vi "is absolute path.vi"(11 "path":string) -> (3 "absolute":bool)   [LabVIEW 2013]
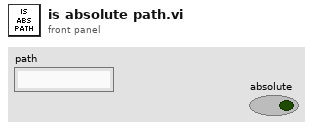
[diagram p1: front panel]
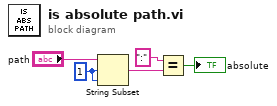
[diagram p0: block diagram]
diagram:
  w2 = 1 ("offset (0)")
  n1 = String Subset(string="path", offset (0)=w2, length (rest)=w2) -> (substring=w3:string)
  n2 = Equal?(x=":", y=w3) -> (x = y?=→"absolute":bool)
